vi "Sub2.vi"(11 "클러스터":T1={{"정지할 차이값"=0.08, "흰색과 밖 차이값"=0.15, "흰/검 반 값 "=0.3}, {"4: 오른각도"=122.0, "4: 뒷쪽각도"=0.0, "5: 오른각도"=120.0, "5: 앞쪽각도"=240.0, "6: 왼쪽각도"=250.0, "6: 앞쪽각도"=128.0}, {"2: 공각도"=233.0, "2: 굴릴각도"=60.0}}) -> ()   [LabVIEW 2014]
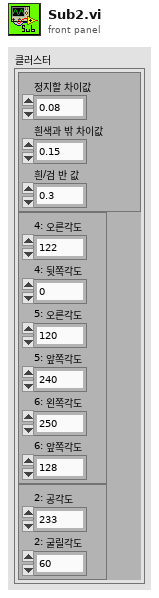
[diagram p1: front panel]
types:
  T1 = cluster{cluster{"정지할 차이값":dbl, "흰색과 밖 차이값":dbl, "흰/검 반 값 ":dbl}, cluster{"4: 오른각도":dbl, "4: 뒷쪽각도":dbl, "5: 오른각도":dbl, "5: 앞쪽각도":dbl, "6: 왼쪽각도":dbl, "6: 앞쪽각도":dbl}, cluster{"2: 공각도":dbl, "2: 굴릴각도":dbl}}
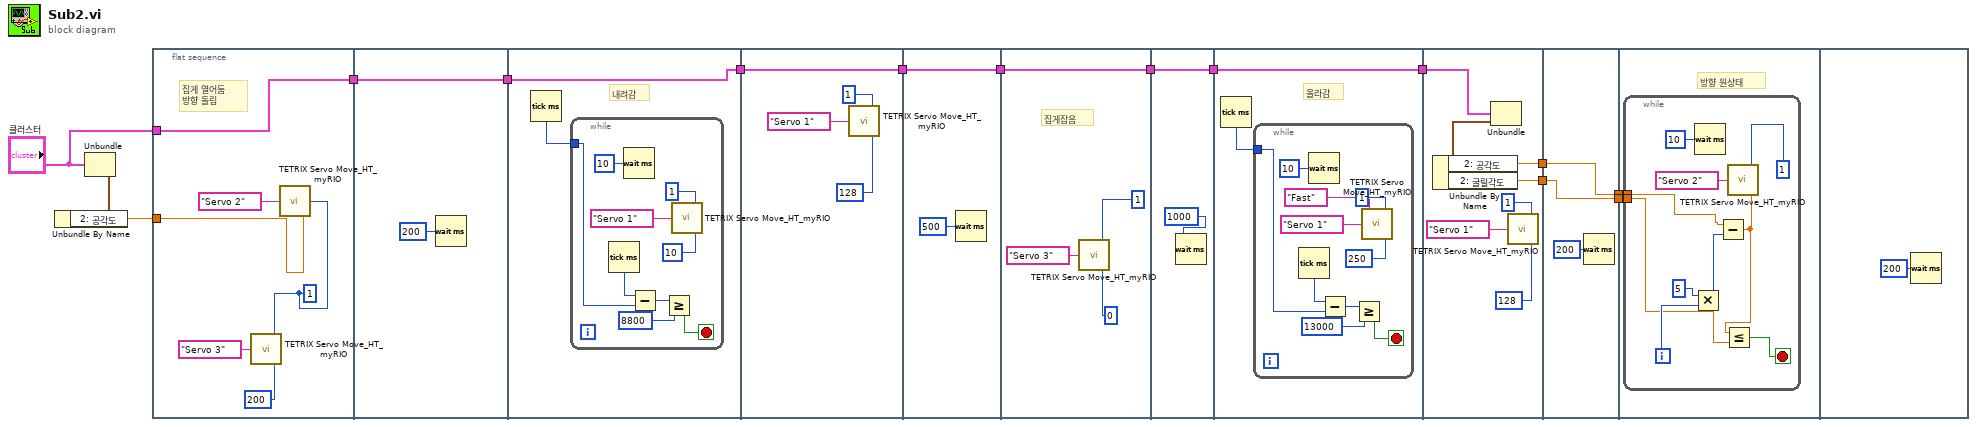
[diagram p0: block diagram]
diagram:
  n1 = Unbundle("클러스터") -> (w15:cluster{"2: 공각도":dbl, "2: 굴릴각도":dbl})  [unwired: 2 out]
  n2 = Unbundle By Name(w15) -> ("2: 공각도"=w14:dbl)
  n3 = flat-sequence {
    tunnel: w14 -> [w17]
    tunnel: [w16] -> w12
    tunnel: "클러스터" -> [w16]
    tunnel: [w22] -> w13
    tunnel: w12 -> [w22]
    tunnel: w13 -> [w24]
    tunnel: [w24] -> w8
    tunnel: [w35] -> w9
    tunnel: w8 -> [w35]
    tunnel: [w39] -> w10
    tunnel: w9 -> [w39]
    tunnel: w10 -> [w41]
    tunnel: [w41] -> w5
    tunnel: [w45] -> w6
    tunnel: w5 -> [w45]
    tunnel: [w47] -> w7
    tunnel: w6 -> [w47]
    tunnel: w7 -> [w62]
    tunnel: [w60] -> w3
    tunnel: [w59] -> w1
    tunnel: [w67] -> w4
    tunnel: w3 -> [w67]
    tunnel: [w66] -> w2
    tunnel: w1 -> [w66]
    tunnel: w4 -> [w70]
    tunnel: w2 -> [w69]
    frame #0 {
      w18 = u8 1 ("Controller Daisy Chain Position (1 - 4)")
      # "집게 열어둠\n방향 돌림"
      n4 = call <vilib>:"TETRIX Servo Move_HT_myRIO.vi"("Servo Position (0 - 255)"=u8 200, "Controller Daisy Chain Position (1 - 4)"=w18, "Select Servo"="Servo 3") -> ()  [unwired: 2 in, 1 out]
      n5 = call <vilib>:"TETRIX Servo Move_HT_myRIO.vi"("Servo Position (0 - 255)"=w17, "Controller Daisy Chain Position (1 - 4)"=w18, "Select Servo"="Servo 2") -> ()  [unwired: 2 in, 1 out]
    }
    frame #1 {
      n6 = Wait (ms)(milliseconds to wait=u32 200 ("대기 시간(ms)")) -> ()  [unwired: 1 out]
    }
    frame #2 {
      # "내려감"
      n7 = Tick Count (ms)() -> (millisecond timer value=w25:u32)
      n8 = while {
        tunnel: w25 -> [w30]
        stop <- w28 stop-if-true
        n9 = Tick Count (ms)() -> (millisecond timer value=w31:u32)
        n10 = Wait (ms)(milliseconds to wait=u32 10 ("대기 시간(ms)")) -> ()  [unwired: 1 out]
        n11 = Subtract(x=w31, y=w30) -> (x-y=w29:u32)
        n12 = Greater Or Equal?(x=w29, y=u32 8800) -> (x >= y?=w28:bool)
        n13 = call <vilib>:"TETRIX Servo Move_HT_myRIO.vi"("Servo Position (0 - 255)"=u8 10, "Controller Daisy Chain Position (1 - 4)"=u8 1, "Select Servo"="Servo 1") -> ()  [unwired: 2 in, 1 out]
      }
    }
    frame #3 {
      n14 = call <vilib>:"TETRIX Servo Move_HT_myRIO.vi"("Servo Position (0 - 255)"=u8 128, "Controller Daisy Chain Position (1 - 4)"=u8 1, "Select Servo"="Servo 1") -> ()  [unwired: 2 in, 1 out]
    }
    frame #4 {
      n15 = Wait (ms)(milliseconds to wait=u32 500 ("대기 시간(ms)")) -> ()  [unwired: 1 out]
    }
    frame #5 {
      # "집게잡음"
      n16 = call <vilib>:"TETRIX Servo Move_HT_myRIO.vi"("Servo Position (0 - 255)"=u8 0, "Controller Daisy Chain Position (1 - 4)"=u8 1, "Select Servo"="Servo 3") -> ()  [unwired: 2 in, 1 out]
    }
    frame #6 {
      n17 = Wait (ms)(milliseconds to wait=u32 1000 ("ms 타이머 값")) -> ()  [unwired: 1 out]
    }
    frame #7 {
      # "올라감"
      n18 = Tick Count (ms)() -> (millisecond timer value=w48:u32)
      n19 = while {
        tunnel: w48 -> [w54]
        stop <- w52 stop-if-true
        n20 = Tick Count (ms)() -> (millisecond timer value=w55:u32)
        n21 = Wait (ms)(milliseconds to wait=u32 10 ("대기 시간(ms)")) -> ()  [unwired: 1 out]
        n22 = Subtract(x=w55, y=w54) -> (x-y=w53:u32)
        n23 = Greater Or Equal?(x=w53, y=u32 13000) -> (x >= y?=w52:bool)
        n24 = call <vilib>:"TETRIX Servo Move_HT_myRIO.vi"("Servo Position (0 - 255)"=u8 250, "Controller Daisy Chain Position (1 - 4)"=u8 1, "Enable Sync: Fast | Medium | Slow | None"="Fast", "Select Servo"="Servo 1") -> ()  [unwired: 1 in, 1 out]
      }
    }
    frame #8 {
      n25 = Unbundle(w62) -> (w61:cluster{"2: 공각도":dbl, "2: 굴릴각도":dbl})  [unwired: 2 out]
      n26 = Unbundle By Name(w61) -> ("2: 공각도"=w60:dbl, "2: 굴릴각도"=w59:dbl)
      n27 = call <vilib>:"TETRIX Servo Move_HT_myRIO.vi"("Servo Position (0 - 255)"=u8 128, "Controller Daisy Chain Position (1 - 4)"=u8 1, "Select Servo"="Servo 1") -> ()  [unwired: 2 in, 1 out]
    }
    frame #9 {
      n28 = Wait (ms)(milliseconds to wait=u32 200 ("대기 시간(ms)")) -> ()  [unwired: 1 out]
    }
    frame #10 {
      # "방향 원상태"
      n29 = while {
        tunnel: w70 -> [w72]
        tunnel: w69 -> [w71]
        i -> [w77]
        stop <- w76 stop-if-true
        n30 = Multiply(x=u8 5 ("Servo Position (0 - 255)"), y=w77) -> (x*y=w75:i32)
        n31 = Wait (ms)(milliseconds to wait=u32 10 ("대기 시간(ms)")) -> ()  [unwired: 1 out]
        n32 = Subtract(x=w72, y=w75) -> (x-y=w74:dbl)
        n33 = Less Or Equal?(x=w74, y=w71) -> (x <= y?=w76:bool)
        n34 = call <vilib>:"TETRIX Servo Move_HT_myRIO.vi"("Servo Position (0 - 255)"=w74, "Controller Daisy Chain Position (1 - 4)"=u8 1, "Select Servo"="Servo 2") -> ()  [unwired: 2 in, 1 out]
      }
    }
    frame #11 {
      n35 = Wait (ms)(milliseconds to wait=u32 200 ("대기 시간(ms)")) -> ()  [unwired: 1 out]
    }
  }
